vi "ActionVIOnCompile.vi"(8 "error in (no error)":errorcluster, 11 "Device Item Ref in":T1 format="%.0x") -> (0 "error out":errorcluster)   [LabVIEW 2016, in "PXImc Custom Device System Explorer.lvlib"]
uses:
  PXImc Custom Device System Explorer.lvlib
  <vilib>/NI Veristand/Custom Device API/Custom Device Item Ref.ctl
  Shared/Compiled.Settings.ctl
  Engine/PXImc Router/Controls/Target Type.ctl
  Engine/PXImc Router/Controls/Router/Router - Config.ctl
  Engine/PXImc Router/Controls/Router/Router - Node Block R-W Properties.ctl
  Engine/PXImc Router/Controls/Router/Router - Block Properties.ctl
  Engine/PXImc Router/Controls/Router/Router - PXImc Properties.ctl
  Engine/PXImc Router/Controls/Router/Router - PXImc Card Properties.ctl
  Engine/PXImc Router/Controls/Node/Node - Config.ctl
  Engine/PXImc Router/Controls/Node/Node - PXImc Parameters.ctl
  Engine/PXImc Router/Controls/Node/Node - Writer Data.ctl
  <vilib>/NI Veristand/VeriStand Data/Byte Buffer/Byte Buffer.lvclass
  Engine/PXImc Router/Controls/Node/Node - Ch Properties.ctl
  Engine/PXImc Router/Controls/Data Type.ctl
  Engine/PXImc Router/Controls/Node/Node - Readers Data.ctl
  Engine/PXImc Router/Controls/Node/Node - Reader Data.ctl
  <vilib>/NI Veristand/Custom Device Tools/Custom Device Utility Library/NI VeriStand - Search for Item by Name.vi
  <vilib>/NI Veristand/Custom Device API/Set Item Property (Variant).vi
  <vilib>/NI VeriStand/Custom Device Tools/Custom Device Utility Library/Custom Device Utility Library.lvlib
  <vilib>/NI VeriStand/Custom Device API/Custom Device API.lvlib
  <vilib>/NI/NIVS Inline Async API/_Data Access System Explorer/Data Access System Explorer.lvlib
  Engine/PXImc Router/PXImc Router.lvlib
  Shared/PXImc Custom Device Shared.lvlib
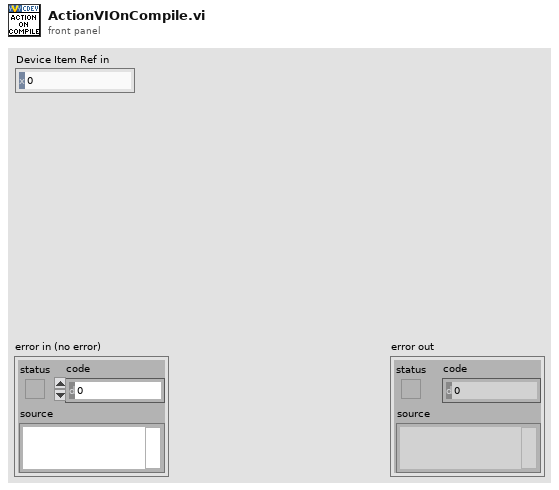
[diagram p1: front panel]
types:
  T1 = typedef "Custom Device API.lvlib/Custom Device Item Ref.ctl" = u64
  T2 = cluster{"Name":string, "Type":enum16{"Output/Write", "Input/Read", "Input/ReadWrite"}, "VS Refs":T1[]}
  T3 = enum16{"Output/Write", "Input/Read", "Input/ReadWrite"}
  T4 = typedef "PXImc Custom Device Shared.lvlib/Compiled.Settings.ctl" = cluster{"Target Type":T5, "Router Properties":T6, "Node Properties":T11}
  T5 = typedef "PXImc Router.lvlib/Target Type.ctl" = enum16{"Router", "Node"}
  T6 = typedef "PXImc Router.lvlib/Router - Config.ctl" = cluster{"Master Table Ref":refnum<data-value>, "Master Table Size (Bytes)":u32, "Nodes Properties":T7[], "Router - PXImc Properties":T9}
  T7 = typedef "PXImc Router.lvlib/Router - Node Block R-W Properties.ctl" = cluster{"Node ID":u32, "# Reading Blocks":u32, "Node Writing Block":T8, "Node Reading Blocks":T8[]}
  T8 = typedef "PXImc Router.lvlib/Router - Block Properties.ctl" = cluster{"Offset":u32, "Size (Bytes)":u32}
  T9 = typedef "PXImc Router.lvlib/Router - PXImc Properties.ctl" = cluster{"PXImc Cards Properties":T10[], "Connection Timeout (s)":dbl, "Readers Buffer Size":u64}
  T10 = typedef "PXImc Router.lvlib/Router - PXImc Card Properties.ctl" = cluster{"PXImc Resource Name":string, "Reader - PXImc Session Ref":refnum<k21>, "Writer - PXImc Session Ref":refnum<k21>, "Reader Conn ID":u16, "Writer Conn ID":u16}
  T11 = typedef "PXImc Router.lvlib/Node - Config.ctl" = cluster{"PXImc Parameters":T12, "Writer Data":T13, "Readers Data":T16}
  T12 = typedef "PXImc Router.lvlib/Node - PXImc Parameters.ctl" = cluster{"Resource Name":string, "Connection Timeout (s)":dbl, "Readers Buffer Size":u64, "Node PXImc Reader Conn Id":u16, "Node PXImc Writer Conn Id":u16, "Writer PXImc Session":refnum<k21>, "Reader PXImc Session":refnum<k21>}
  T13 = typedef "PXImc Router.lvlib/Node - Writer Data.ctl" = cluster{"Noder ID":u32, "Byte Buffer Ref":refnum<class "Byte Buffer.lvclass">, "Master Table Offest":u32, "Byte Buffer Size":u32, "Node Local Channels":T14[]}
  T14 = typedef "PXImc Router.lvlib/Node - Ch Properties.ctl" = cluster{"Value":dbl, "Data Type":T15}
  T15 = typedef "PXImc Router.lvlib/Data Type.ctl" = enum16{"Boolean", "SGL", "DBL", "I8", "I16", "I32", "I64", "U8", "U16", "U32", "U64"}
  T16 = typedef "PXImc Router.lvlib/Node - Readers Data.ctl" = cluster{"Byte Buffer Ref":refnum<class "Byte Buffer.lvclass">, "Byte Buffer Size":u64, "Readers Data Array":T17[]}
  T17 = typedef "PXImc Router.lvlib/Node - Reader Data.ctl" = cluster{"Noder ID":u32, "Master Table Offest":u32, "Byte Buffer Size":u64, "Node Local Channels":T14[]}
  T18 = typedef "Custom Device API.lvlib/Custom Device Item Info.ctl" = cluster{"Name":string, "Is Channel":bool, "GUID":string, "Is Waveform":bool}
  T19 = cluster{"Name":string, "Type":enum16{"Output/Write", "Input/Read", "Input/ReadWrite"}, "VS Refs":T1[]}[]
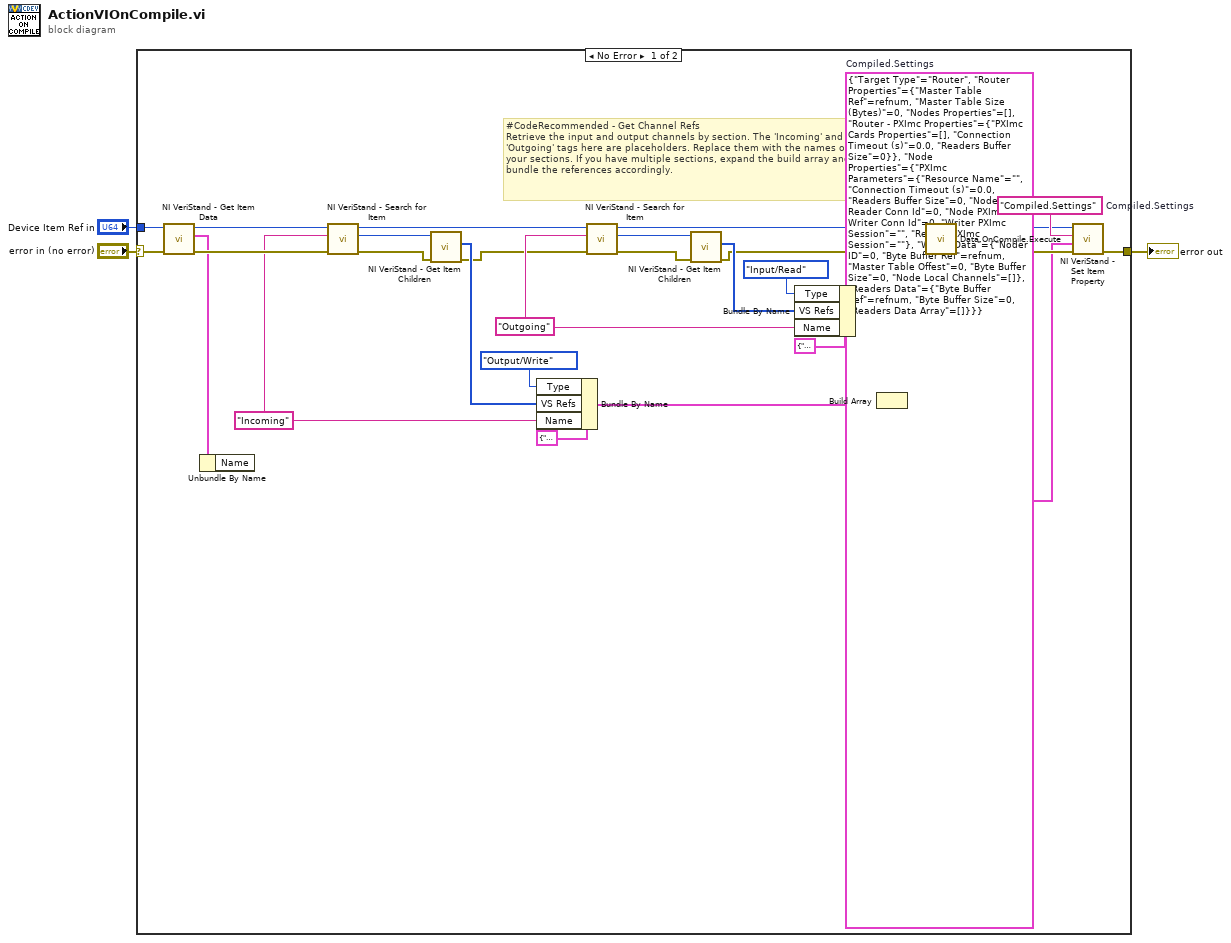
[diagram p0: block diagram]
diagram:
  n1 = case shown="No Error" "error in (no error)" {
    selector: "error in (no error)" -> [w26 w33]
    tunnel: [w27 w33] -> w2
    tunnel: "Device Item Ref in" -> [w25 _]
    frame No Error {
      w4 = T4 {"Target Type"=enum."Router", "Router Properties"={"Master Table Ref"=refnum, "Master Table Size (Bytes)"=0, "Nodes Properties"=[], "Router - PXImc Properties"={"PXImc Cards Properties"=[], "Connection Timeout (s)"=0.0, "Readers Buffer Size"=0}}, "Node Properties"={"PXImc Parameters"={"Resource Name"="", "Connection Timeout (s)"=0.0, "Readers Buffer Size"=0, "Node PXImc Reader Conn Id"=0, "Node PXImc Writer Conn Id"=0, "Writer PXImc Session"="", "Reader PXImc Session"=""}, "Writer Data"={"Noder ID"=0, "Byte Buffer Ref"=refnum, "Master Table Offest"=0, "Byte Buffer Size"=0, "Node Local Channels"=[]}, "Readers Data"={"Byte Buffer Ref"=refnum, "Byte Buffer Size"=0, "Readers Data Array"=[]}}}  # Compiled.Settings
      w19 = "Outgoing" ("Item Name")
      w21 = "Incoming" ("Item Name")
      w28 = "Compiled.Settings"  # Compiled.Settings
      # "#CodeRecommended - Get Channel Refs\nRetrieve the input and output channels by section. The 'Incoming' and 'Outgoing' tags here are placeholders. Replace them with the names of your sections. If you have multiple sections, expand the build array and bundle the references accordingly."
      n2 = call <vilib>:"NI VeriStand - Get Item Data.vi"("error in (no error)"=w26, "Item Ref in"=w25) -> ("error out"=w23:errorcluster, "Item Info"=w22:T18, "Item Ref out"=w24:T1)  [unwired: 6 in, 1 out]
      n3 = Unbundle By Name(w22) -> ()  [unwired: 1 out]
      n4 = call-poly <vilib>:"NI VeriStand - Search for Item.vi"("error in"=w23, "Item Name"=w21, "Section Ref in"=w24) -> ("error out"=w32:errorcluster, "Item Ref"=w31:T1, "Section Ref out"=w8:T1)  [unwired: 5 in, 1 out]
      n5 = call <vilib>:"NI VeriStand - Get Item Children.vi"("error in (no error)"=w32, "Item Ref in"=w31) -> ("error out"=w7:errorcluster, "Child Refs"=w20:T1[])  [unwired: 6 in, 2 out]
      n6 = Bundle By Name(cluster=T2 {"Name"="", "Type"=enum."Output/Write", "VS Refs"=[]} ("Group"), "Type"=T3."Output/Write", "VS Refs"=w20, "Name"=w21) -> (w11:T2)
      n7 = call-poly <vilib>:"NI VeriStand - Search for Item.vi"("error in"=w7, "Item Name"=w19, "Section Ref in"=w8) -> ("error out"=w29:errorcluster, "Item Ref"=w30:T1, "Section Ref out"=w9:T1)  [unwired: 5 in, 1 out]
      n8 = call <vilib>:"NI VeriStand - Get Item Children.vi"("error in (no error)"=w29, "Item Ref in"=w30) -> ("error out"=w10:errorcluster, "Child Refs"=w15:T1[])  [unwired: 6 in, 2 out]
      n9 = Bundle By Name(cluster=T2 {"Name"="", "Type"=enum."Output/Write", "VS Refs"=[]} ("Group"), "Type"=T3."Input/Read", "VS Refs"=w15, "Name"=w19) -> (w17:T2)
      n10 = Build Array(w17, w11) -> (w14:T19)
      n11 = call <vilib>:"Data.OnCompile.Execute.vi"("error in"=w10, "VS Ref Groups"=w14, "Custom Device Ref"=w9) -> ("error out"=w6:errorcluster, "Custom Device Ref"=w5:T1)  [unwired: 7 in]
      n12 = call-poly <vilib>:"NI VeriStand - Set Item Property.vi"("error in (no error)"=w6, "Value"=w4, "Property Name"=w28, "Item Ref in"=w5) -> ("error out"=w27:errorcluster)  [unwired: 5 in, 2 out]
    }
    frame Error {
    }
  }
  "error out" <- w2
